vi "Endpoint Connected.vi"(8 "error in (no error)":errorcluster, 10 "Endpoint":refnum<class "Message Enqueuer.lvclass">, 11 "Nested Endpoint Caller in":refnum<class "Nested Endpoint Caller.lvclass">) -> (0 "error out":errorcluster, 3 "Nested Endpoint Caller out":refnum<class "Nested Endpoint Caller.lvclass">)   [LabVIEW 2020, in "Nested Endpoint Caller.lvlib" / "Nested Endpoint Caller.lvclass"]
doc: "Override this method to specify how the receiving actor responds to a Connected message from a nested endpoint actor."
uses:
  Nested Endpoint Caller.lvclass
  <vilib>/ActorFramework/Message Enqueuer/Message Enqueuer.lvclass
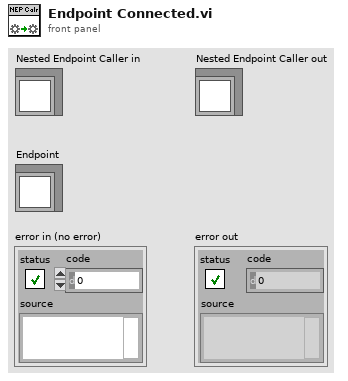
[diagram p1: front panel]
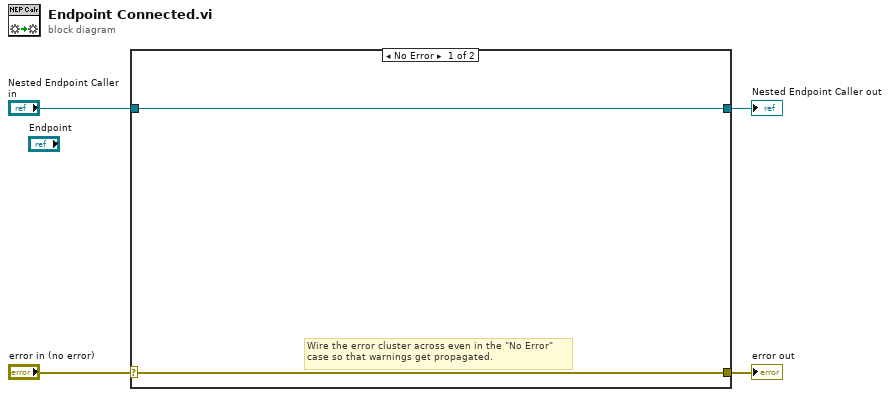
[diagram p0: block diagram]
diagram:
  n1 = case shown="No Error" "error in (no error)" {
    selector: "error in (no error)" -> [w5 w8]
    tunnel: [w5 w8] -> w3
    tunnel: [w6 w7] -> w1
    tunnel: "Nested Endpoint Caller in" -> [w6 w7]
    frame No Error {
      # "Wire the error cluster across even in the \"No Error\"\ncase so that warnings get propagated."
    }
    frame Error {
    }
  }
  "error out" <- w3
  "Nested Endpoint Caller out" <- w1
